vi "19 - Joysticks.vi"() -> ()   [LabVIEW 2019]
uses:
  Libraries/LibSDL2 Wrapper/Controls/Keyboard Event.ctl
  Libraries/LibSDL2 Wrapper/Controls/Mouse Motion Event.ctl
  Libraries/LibSDL2 Wrapper/Controls/Mouse Button Event.ctl
  Libraries/LibSDL2 Wrapper/Controls/Joysitck Axis Event.ctl
  Libraries/LibSDL2 Wrapper/Controls/Joysitck Button Event.ctl
  Libraries/LibSDL2 Wrapper/Controls/Joysitck Hat Event.ctl
  Libraries/LibSDL2 Wrapper/Controls/Joystick Hat Value.ctl
  Libraries/LibSDL2 Wrapper/Controls/Init Flags.ctl
  Libraries/LibSDL2 Wrapper/LibSDL2.lvlib
panel:
  out "Joystick Hat Event":T1 {"Which" format="%.0x"; "Type" format="%.0x"}
  out "Buttons":bool[](array[boolean])
  out "Joystick Button Event":T3 {"State" format="%.0x"; "Which" format="%.0x"; "Type" format="%.0x"}
  out "R Trigger":i32(slide) scale=-33000.0..33000.0
  out "R Trigger":i32(slide) scale=-33000.0..33000.0
  out "R Stick X":i32(slide) scale=-33000.0..33000.0
  out "L Trigger":i32(slide) scale=-33000.0..33000.0
  out "L Stick Y":i32(slide) scale=-33000.0..33000.0
  out "L Stick X":i32(slide) scale=-33000.0..33000.0
  out "Axes":i16[](array[numeric])
  out "Joystick Axis Event":T4 {"Padding 4" format="%.0x"; "Value" format="%.0x"; "Padding 3" format="%.0x"; "Padding 2" format="%.0x"; "Which" format="%.0x"; "Type" format="%.0x"}
  out "Number Of Joysticks":i32
  out "Iteration":i32
  out "Loop Period [s]":dbl format="%.1p"
  out "Event Type":u32 format="%.0x"
  out "Mouse Button Event":T5
  out "Mouse Motion Event":T6
  out "Keyboard Event":T7 {"Padding 2" format="%.0x"; "Padding 1" format="%.0x"; "Window ID" format="%.0x"; "Type" format="%.0x"; "Key Sym"."Unused" format="%.0x"; "Key Sym"."Mod" format="%.0x"; "Key Sym"."Sym" format="%.0x"; "Key Sym"."Scan Code" format="%.0x"}
  out "Error":string
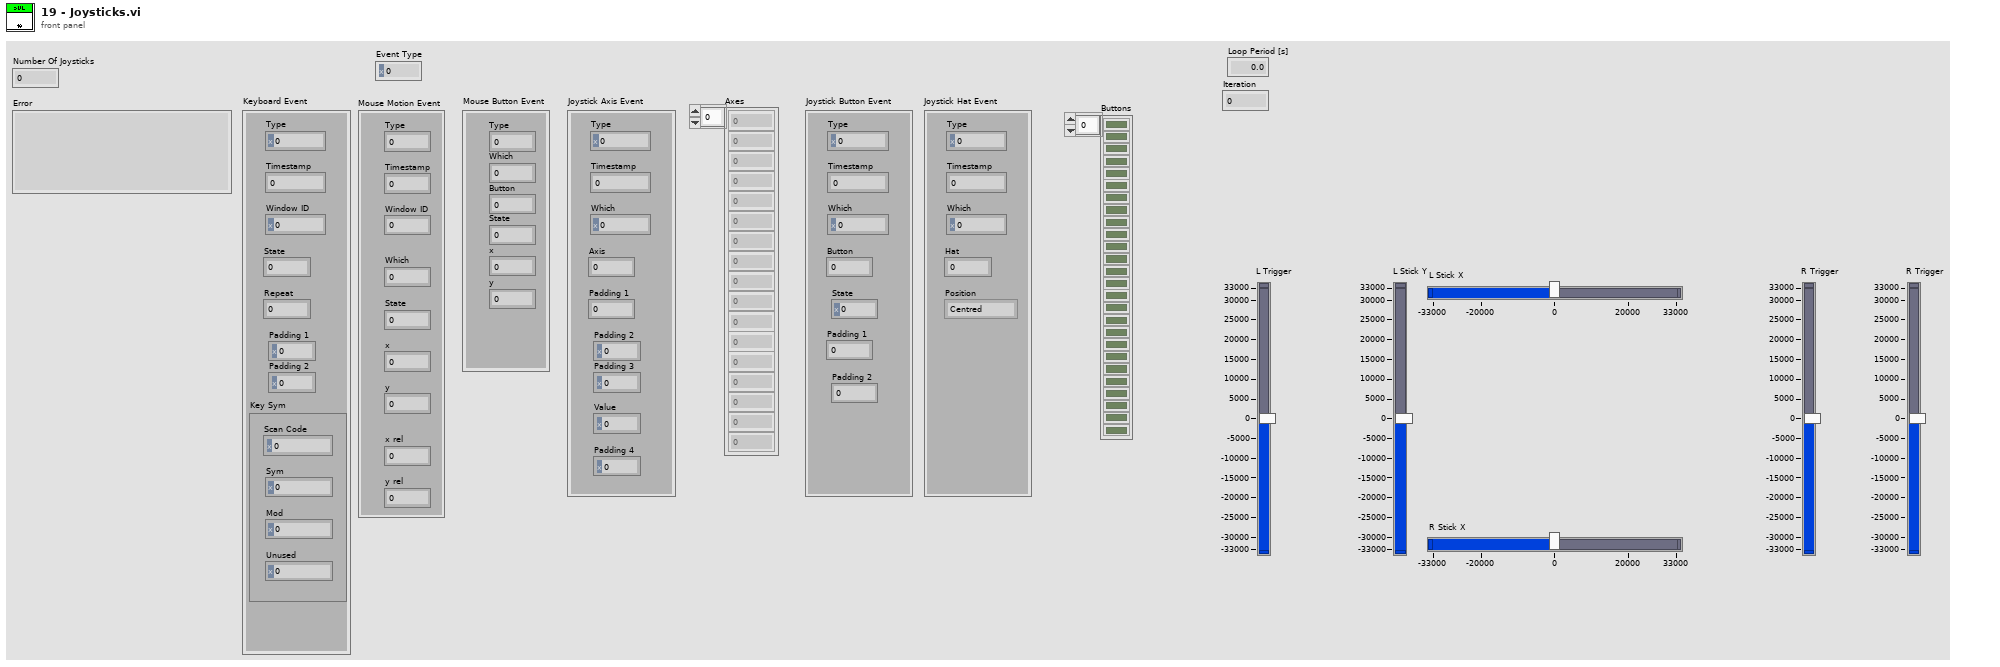
[diagram p1: front panel]
types:
  T1 = typedef "LibSDL2.lvlib/Joysitck Hat Event.ctl" = cluster{"Type":u32, "Timestamp":u32, "Which":i32, "Hat":u8, "Position":T2}
  T2 = typedef "LibSDL2.lvlib/Joystick Hat Value.ctl" = enum16{"Centred", "Up", "Right", "Down", "Left", "Right Up", "Right Down", "Left Up", "Left Down"}
  T3 = typedef "LibSDL2.lvlib/Joysitck Button Event.ctl" = cluster{"Type":u32, "Timestamp":u32, "Which":i32, "Button":u8, "State":u8, "Padding 1":u8, "Padding 2":u8}
  T4 = typedef "LibSDL2.lvlib/Joysitck Axis Event.ctl" = cluster{"Type":u32, "Timestamp":u32, "Which":i32, "Axis":u8, "Padding 1":u8, "Padding 2":u8, "Padding 3":u8, "Value":i16, "Padding 4":u16}
  T5 = typedef "LibSDL2.lvlib/Mouse Button Event.ctl" = cluster{"Type":u8, "Which":u8, "Button":u8, "State":u8, "x":u16, "y":u16}
  T6 = typedef "LibSDL2.lvlib/Mouse Motion Event.ctl" = cluster{"Type":u32, "Timestamp":u32, "Window ID":u32, "Which":u32, "State":u32, "x":i32, "y":i32, "x rel":i32, "y rel":i32}
  T7 = typedef "LibSDL2.lvlib/Keyboard Event.ctl" = cluster{"Type":u32, "Timestamp":u32, "Window ID":u32, "State":u8, "Repeat":u8, "Padding 1":u8, "Padding 2":u8, "Key Sym":cluster{"Scan Code":u32, "Sym":i32, "Mod":u16, "Unused":u32}}
  T8 = typedef "LibSDL2.lvlib/Init Flags.ctl" = u32
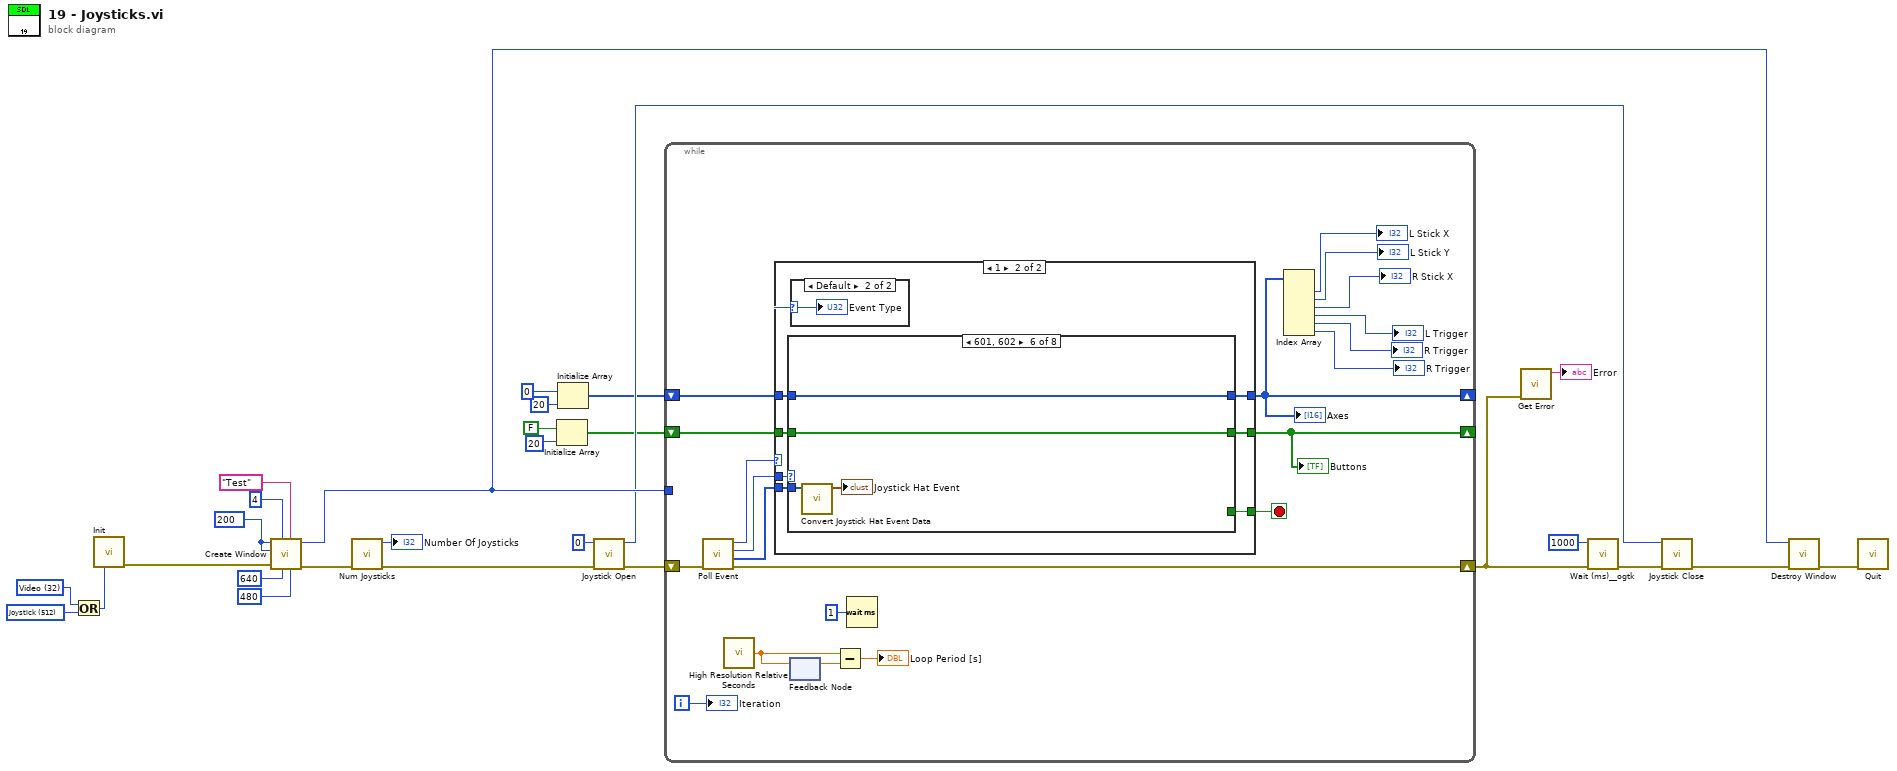
[diagram p0: block diagram]
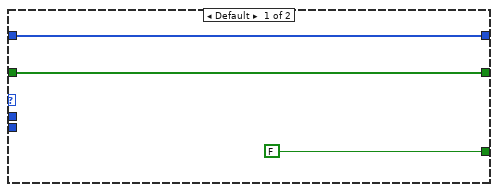
[diagram p2: hidden frame]
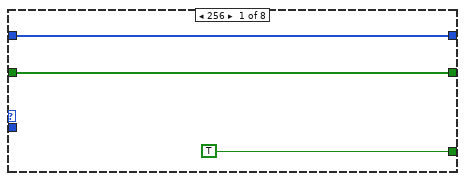
[diagram p4: hidden frame]
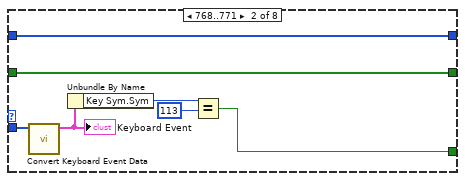
[diagram p5: hidden frame]
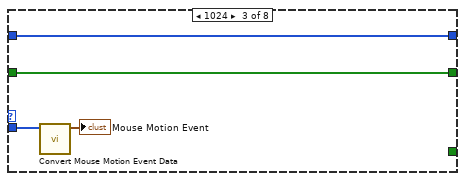
[diagram p6: hidden frame]
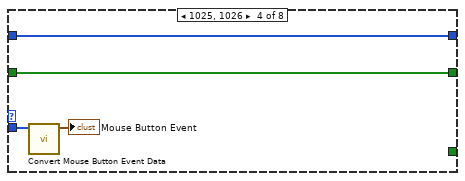
[diagram p7: hidden frame]
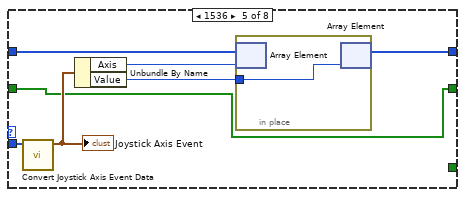
[diagram p8: hidden frame]
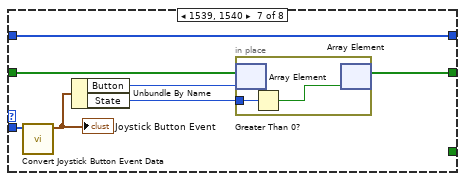
[diagram p9: hidden frame]
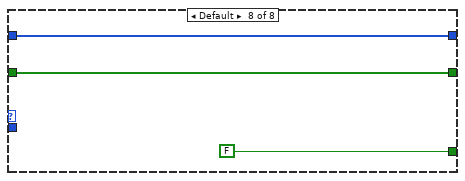
[diagram p10: hidden frame]
diagram:
  w18 = T8 512 items=["Timer"=1, "Audio"=16, "Video"=32, "Joystick"=512, "Haptic"=4096, "Game Controller"=8192, "Events"=16384, "No Parachute"=1048576, "Everything"=17244689] ("Init Flags")
  w15 = T8 32 items=["Timer"=1, "Audio"=16, "Video"=32, "Joystick"=512, "Haptic"=4096, "Game Controller"=8192, "Events"=16384, "No Parachute"=1048576, "Everything"=17244689] ("Init Flags")
  w1 = u32 200 ("Flags")
  n1 = Or(x=w15, y=w18) -> (x .or. y?=w14:T8)
  n2 = call "Init.vi"("Flags"=w14) -> ("error out"=w25:errorcluster)  [unwired: 9 in, 1 out]
  n3 = call "Create Window.vi"("Height"=480, "Title"="Test", "Width"=640, "Flags"=u32 4, "error in"=w25, "Position y"=w1, "Position x"=w1) -> ("error out"=w17:errorcluster, "Window Pointer"=w19:u32)  [unwired: 3 in]
  n4 = call "Num Joysticks.vi"("error in"=w17) -> ("error out"=w13:errorcluster, "Number Of Joysticks"=→"Number Of Joysticks":i32)  [unwired: 9 in]
  n5 = Initialize Array(FALSE, 20 ("dimension size")) -> (w2:bool[])
  n6 = Initialize Array(i16 0, 20 ("dimension size")) -> (w7:i16[])
  n7 = call "Joystick Open.vi"("error in"=w13, "Device Index"=0) -> ("error out"=w12:errorcluster, "Joystick Pointer"=w8:u32)  [unwired: 8 in]
  n8 = while {
    tunnel: w19 -> [_]
    shift-right: [w42] -> w20
    shift-left: w12 -> [w49]
    shift-right: [w37] -> _
    shift-left: w7 -> [w38]
    shift-right: [w31] -> _
    shift-left: w2 -> [w32]
    i -> [w41]
    stop <- w47 stop-if-true
    n9 = call "Poll Event.vi"("error in"=w49) -> ("error out"=w42:errorcluster, "Event Data"=w48:u8[], "Event Type"=w46:u32, "Return"=w40:i32)  [unwired: 7 in]
    n10 = call <vilib>:"High Resolution Relative Seconds.vi"() -> ("relative seconds"=w45:dbl)
    n11 = case shown="1" w40 {
      tunnel: w48 -> [_ w59]
      tunnel: [FALSE w58] -> w47
      tunnel: w46 -> [_ w57]
      tunnel: w38 -> [w51 w56]
      tunnel: [w51 w55] -> w37
      tunnel: w32 -> [w50 w54]
      tunnel: [w50 w53] -> w31
      frame Default {
      }
      frame 1 {
        n12 = case shown="601, 602" w57 {
          tunnel: w59 -> [_ w70 w74 w78 w85 w90 w97 _]
          tunnel: [TRUE w66 _ _ _ _ _ FALSE] -> w58
          tunnel: w56 -> [w62 w65 w72 w76 w83 w87 w91 w101]
          tunnel: [w62 w65 w72 w76 w80 w87 w91 w101] -> w55
          tunnel: w54 -> [w61 w64 w71 w75 w79 w89 w93 w100]
          tunnel: [w61 w64 w71 w75 w79 w89 w92 w100] -> w53
          frame 256 {
          }
          frame 768..771 {
            n13 = call "Convert Keyboard Event Data.vi"("Event Data"=w70) -> ("Keyboard Event"=w69:T7)  [unwired: 10 in]
            "Keyboard Event" <- w69
            n14 = Unbundle By Name(w69) -> ("Key Sym.Sym"=w68:i32)
            n15 = Equal?(x=w68, y=113) -> (x = y?=w66:bool)
          }
          frame 1024 {
            n16 = call "Convert Mouse Motion Event Data.vi"("Event Data"=w74) -> ("Mouse Motion Event"=→"Mouse Motion Event":T6)  [unwired: 10 in]
          }
          frame 1025, 1026 {
            n17 = call "Convert Mouse Button Event Data.vi"("Event Data"=w78) -> ("Mouse Button Event"=→"Mouse Button Event":T5)  [unwired: 10 in]
          }
          frame 1536 {
            n18 = call "Convert Joystick Axis Event Data.vi"("Event Data"=w85) -> ("Joystick Axis Event"=w84:T4)  [unwired: 10 in]
            "Joystick Axis Event" <- w84
            n19 = Unbundle By Name(w84) -> ("Axis"=w82:u8, "Value"=w81:i16)
            n20 = in-place {
              in-place-border: w81 -> [w86]
              n21 = in-place-array #1(w83, w82) -> ()  [unwired: 1 out]
              n22 = in-place-array #1(w86) -> (w80:i16[])  [unwired: 1 out]
            }
          }
          frame 1537, 1538 {
            n23 = call "Convert Joystick Hat Event Data.vi"("Event Data"=w90) -> ("Joystick Hat Event"=→"Joystick Hat Event":T1)  [unwired: 10 in]
          }
          frame 1539, 1540 {
            n24 = call "Convert Joystick Button Event Data.vi"("Event Data"=w97) -> ("Joystick Button Event"=w96:T3)  [unwired: 10 in]
            "Joystick Button Event" <- w96
            n25 = Unbundle By Name(w96) -> ("Button"=w95:u8, "State"=w94:u8)
            n26 = in-place {
              in-place-border: w94 -> [w99]
              n27 = in-place-array #2(w93, w95) -> ()  [unwired: 1 out]
              n28 = Greater Than 0?(x=w99) -> (x > 0?=w98:bool)
              n29 = in-place-array #2(w98) -> (w92:bool[])  [unwired: 1 out]
            }
          }
          frame Default {
          }
        }
        n30 = case shown="Default" w57 {
          selector: w57 -> [_ w60]
          frame 0 {
          }
          frame Default {
            "Event Type" <- w60
          }
        }
      }
    }
    "Axes" <- w37
    "Buttons" <- w31
    n31 = feedback-in #3(w45) -> ()
    n32 = feedback #3() -> (w44:dbl)  [unwired: 1 in]
    n33 = Subtract(x=w45, y=w44) -> (x-y=→"Loop Period [s]":dbl)
    n34 = Wait (ms)(milliseconds to wait=u32 1) -> ()  [unwired: 1 out]
    n35 = Index Array(array=w37) -> (element #1=→"L Stick X":i16, element #2=→"L Stick Y":i16, element #3=→"R Stick X":i16, element #4=→"L Trigger":i16, element #5=→"R Trigger":i16, element #6=→"R Trigger":i16)  [unwired: 6 in]
    "Iteration" <- w41
  }
  n36 = call "Get Error.vi"("error in"=w20) -> ("Error"=→"Error":string)  [unwired: 9 in, 1 out]
  n37 = call <userlib>:"Wait (ms)__ogtk.vi"("error in (no error)"=w20, "milliseconds to wait"=u32 1000) -> ("error out"=w10:errorcluster)  [unwired: 8 in, 1 out]
  n38 = call "Joystick Close.vi"("error in"=w10, "Joystick Pointer"=w8) -> ("error out"=w9:errorcluster)  [unwired: 9 in]
  n39 = call "Destroy Window.vi"("error in"=w9, "Window Pointer"=w19) -> ("error out"=w22:errorcluster)  [unwired: 9 in]
  n40 = call "Quit.vi"("error in"=w22) -> ()  [unwired: 10 in, 1 out]
